vi "waitOnIRQ.vi"(8 "error in (no error)":errorcluster, 10 "Timeout (ms)":i32, 11 "Subnet in":refnum<class "Subnet.lvclass">) -> (0 "error out":errorcluster, 3 "Subnet out":refnum<class "Subnet.lvclass">)   [LabVIEW 2016, in "Subnet.lvclass"]
uses:
  Subnet.lvclass
  Subnet.lvclass/Subnet.ctl
  Common_RT_Modbus/IModbus/IModbus.lvclass
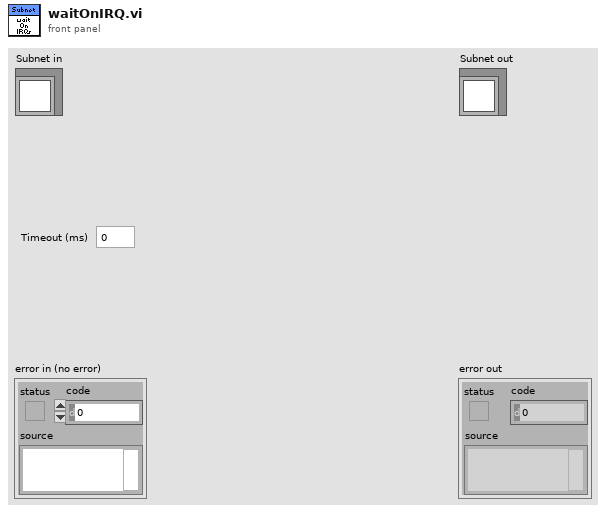
[diagram p1: front panel]
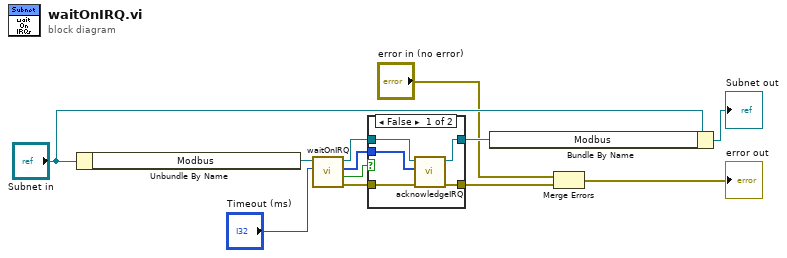
[diagram p0: block diagram]
diagram:
  n1 = Unbundle By Name("Subnet in") -> ("Modbus"=w1:refnum<class "IModbus.lvclass">)
  n2 = call-dynamic "waitOnIRQ.vi"("Timeout"="Timeout (ms)", "IModbus in"=w1) -> ("error out"=w7:errorcluster, "TimedOut"=w11:bool, "IRQs"=w6:i32[], "IModbus out"=w10:refnum<class "IModbus.lvclass">)  [unwired: 6 in]
  n3 = case shown="False" w11 {
    tunnel: w10 -> [w17 w19]
    tunnel: [w16 w19] -> w8
    tunnel: w7 -> [w15 w18]
    tunnel: w6 -> [w14 _]
    tunnel: [w13 w18] -> w5
    frame False {
      n4 = call-dynamic "acknowledgeIRQ.vi"("error in (no error)"=w15, "IRQs"=w14, "IModbus in"=w17) -> ("error out"=w13:errorcluster, "IModbus out"=w16:refnum<class "IModbus.lvclass">)  [unwired: 7 in]
    }
    frame True {
    }
  }
  n5 = Bundle By Name(cluster="Subnet in", "Modbus"=w8) -> (→"Subnet out":refnum<class "Subnet.lvclass">)
  n6 = Merge Errors("error in (no error)", w5) -> (→"error out":errorcluster)
